vi "Get Datalogger.vi"(8 "error in (no error)":errorcluster, 11 "Base Step in":refnum<class "Base Step.lvclass">) -> (0 "error out":errorcluster, 2 "Datalogger":refnum<class "Datalogger.lvclass">, 3 "Base Step out":refnum<class "Base Step.lvclass">)   [LabVIEW 2020]
uses:
  Classes/Datalogger/Datalogger.lvclass
  Base Step.lvclass
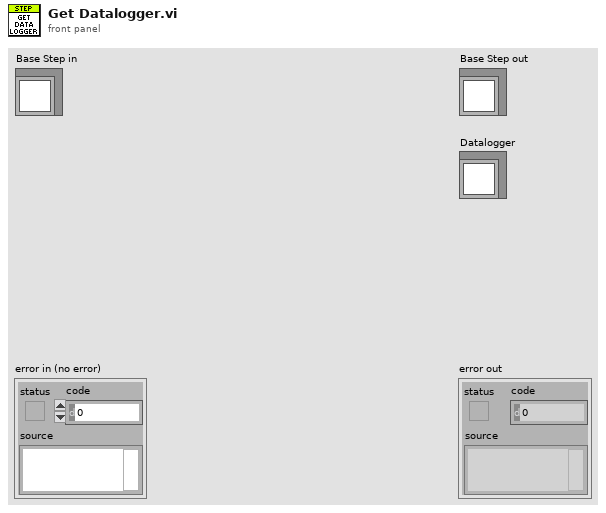
[diagram p1: front panel]
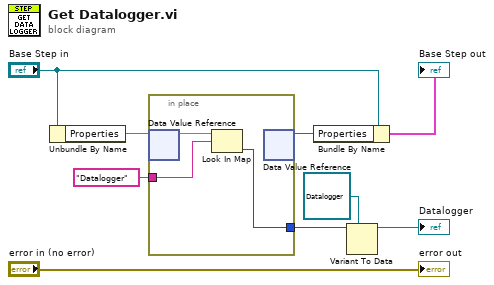
[diagram p0: block diagram]
diagram:
  n1 = Unbundle By Name("Base Step in") -> ("Properties"=w6)
  n2 = in-place {
    in-place-border: "Datalogger" ("Key") -> [w12]
    in-place-border: [w10] -> w3
    n3 = in-place-dvr #1(w6) -> (w11:dbl)  [unwired: 1 out]
    n4 = Look In Map(map=w11, key=w12) -> (value=w10:i32)  [unwired: 1 in, 1 out]
    n5 = in-place-dvr #1() -> (w5:refnum<data-value>)  [unwired: 1 in, 1 out]
  }
  n6 = Bundle By Name(cluster="Base Step in", "Properties"=w5) -> (→"Base Step out":cluster{})
  n7 = Variant To Data(type=refnum<class "Datalogger.lvclass"> refnum ("Datalogger"), Variant=w3) -> (data=→"Datalogger":refnum<class "Datalogger.lvclass">)  [unwired: 1 in, 1 out]
  "error out" <- "error in (no error)"
